vi "Sensor Data.vi"   [LabVIEW 2020, in "Lake Shore 336.lvlib"]
uses:
  Lake Shore 336.lvlib
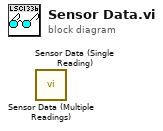
[diagram p0: block diagram]
diagram:
  n1 = call "Sensor Data (Multiple Readings).vi"() -> ()  [unwired: 9 in, 3 out]
  n2 = call "Sensor Data (Single Reading).vi"() -> ()  [unwired: 9 in, 3 out]
